vi "IMU Loop.vi"(8 "error in (no error)":errorcluster, 11 "FPGA ref in":refnum<k20>) -> (0 "error out":errorcluster)   [LabVIEW 2016]
uses:
  Typedef/INS Data.ctl
  <vilib>/Utility/error.llb/Error Cluster From Error Code.vi
  <vilib>/RVI Host/nirviSupport.llb/nirviErrorClusterFromErrorCode.vi
  <vilib>/rvi/errors/niLvFpgaAdjustHostInterfaceError.vi
  <vilib>/rvi/interface/nirviMethod/nirviMethod.xnode
  <vilib>/ErrorRing/Error Ring.xnode
  <vilib>/rvi/interface/nirviMethod/StockFPGA_InlinedMethodWaitForSingleIRQ.vi
  <vilib>/FPGAPlugInAG/Dynamic/niLvFpga_WaitOnIrq_Dynamic.vi
  <vilib>/FPGAPlugInAG/Dynamic/niLvFpga_AcknowledgeIrq_Dynamic.vi
panel:
  out "FPGA ref Out":refnum<k20>
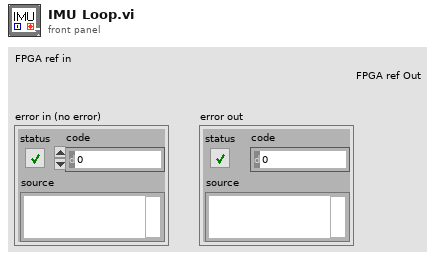
[diagram p1: front panel]
types:
  T1 = typedef "INS Data.ctl" = cluster{"Yaw":sgl, "Pitch":sgl, "Roll":sgl, "Lat":dbl, "Long":dbl, "Alt":dbl, "North":dbl, "East":dbl, "Down":dbl, "PosU":dbl, "VelU":dbl}
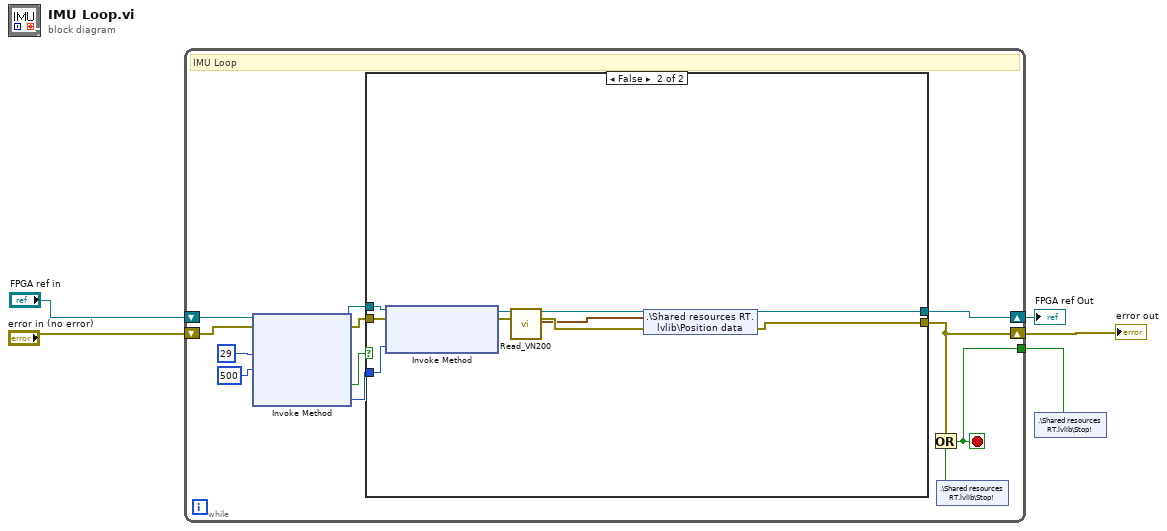
[diagram p0: block diagram]
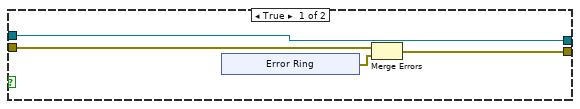
[diagram p2: hidden frame]
diagram:
  n1 = while {
    shift-right: [w15] -> w2
    shift-left: "error in (no error)" -> [w13]
    shift-right: [w17] -> w1
    shift-left: "FPGA ref in" -> [w12]
    tunnel: [w14] -> w3
    stop <- w14 stop-if-true
    # "IMU Loop"
    n2 = xnode "Invoke Method"("FPGA VI Reference In"=w12, "error in"=w13, "IRQ Number(s)"=29, "Timeout (ms)"=500) -> ("FPGA VI Reference Out"=w7:refnum<k20>, "error out"=w8:errorcluster, "Timed Out"=w9:bool, "IRQ(s) Asserted"=w6:i32)
    n3 = case shown="False" w9 {
      tunnel: w8 -> [w20 w29]
      tunnel: w7 -> [w21 w33]
      tunnel: [w21 w35] -> w17
      tunnel: [w19 w30] -> w15
      tunnel: w6 -> [_ w31]
      frame True {
        n4 = xnode "Error Ring"() -> ("error out"=w18:errorcluster)
        n5 = Merge Errors(w20, w18) -> (w19:errorcluster)
      }
      frame False {
        n6 = xnode "Invoke Method"("FPGA VI Reference In"=w33, "error in"=w29, "IRQ Number(s)"=w31) -> ("FPGA VI Reference Out"=w28:refnum<k20>, "error out"=w32:errorcluster)
        n7 = call "Read_VN200.vi"("FPGA Interface"=w28, "error in"=w32) -> ("FPGA Interface Out"=w35:refnum<k20>, "error out"=w34:errorcluster, "Position Data"=w27:T1)  [unwired: 11 in]
        n8 = shared-variable ".\\Shared resources RT.lvlib\\Position data"(w27, error in=w34) -> (error out=w30:errorcluster)
      }
    }
    n9 = shared-variable ".\\Shared resources RT.lvlib\\Stop!"() -> (w16:bool)  [unwired: 1 in, 1 out]
    n10 = Or(x=w15, y=w16) -> (x .or. y?=w14:bool)
  }
  "error out" <- w2
  "FPGA ref Out" <- w1
  n11 = shared-variable ".\\Shared resources RT.lvlib\\Stop!"(w3) -> ()  [unwired: 1 in, 1 out]
